vi "SequenceEditor.vi"() -> ()   [LabVIEW 2017]
panel:
  in  "Properties Table":refnum<k24>(container)
  out "IsBusy":bool=TRUE
  out "ExpID":string="Exp967f258c607eed45caf40f4c3101458dC" caption="Exp. ID (Debug)"
  out "Reduced Sequence":dbl[](graph)
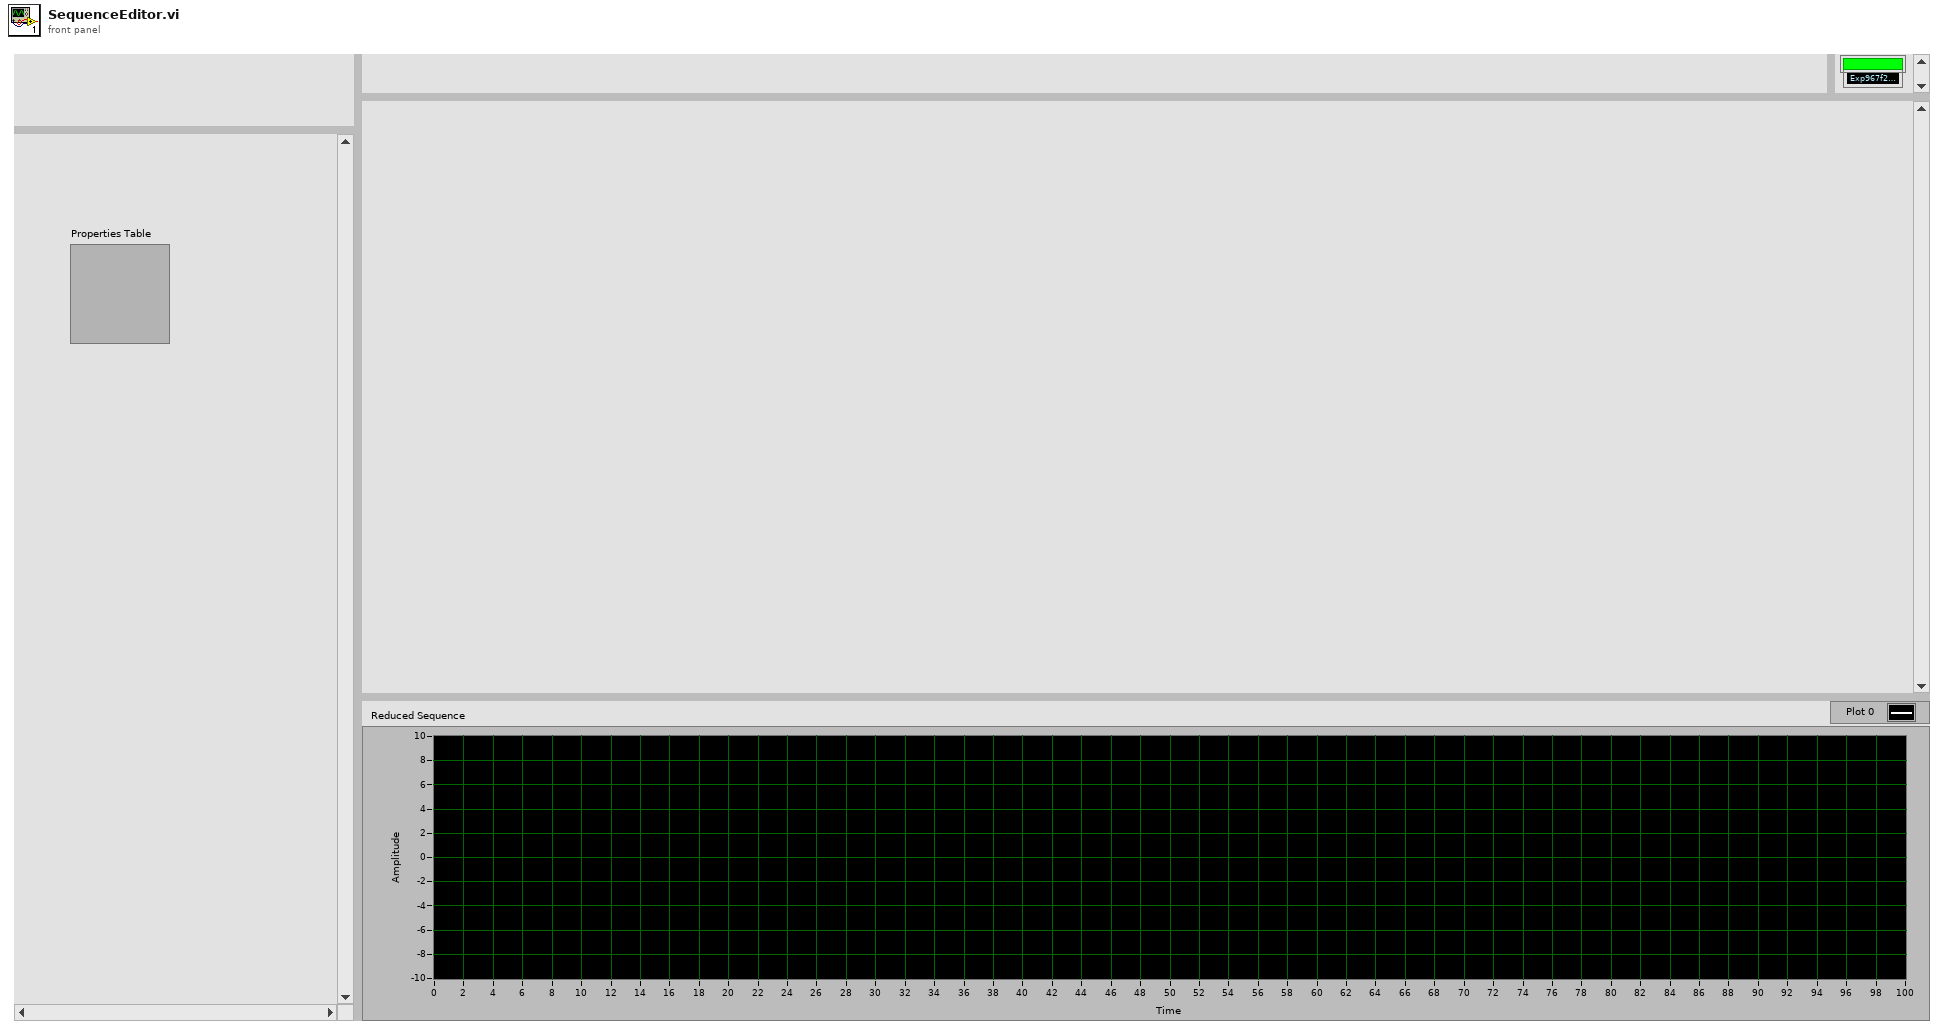
[diagram p1: front panel]
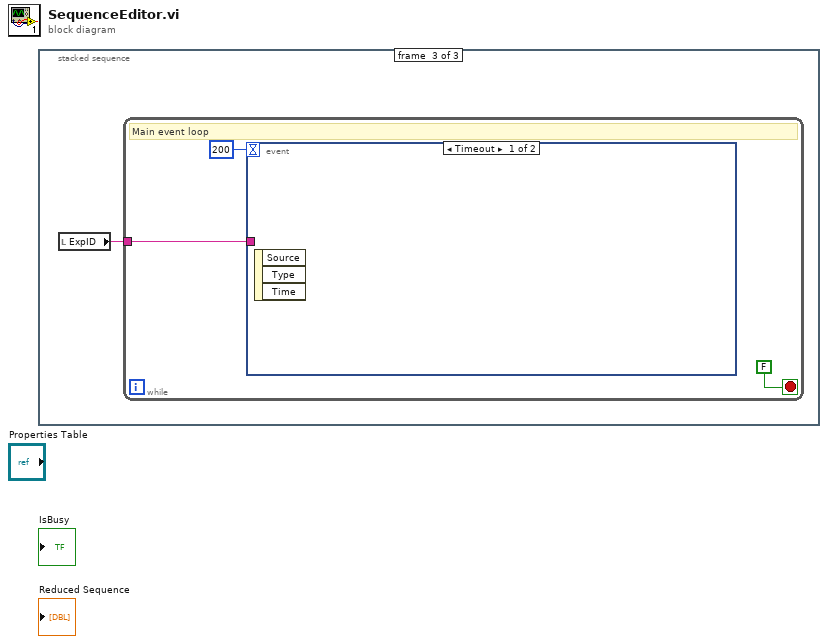
[diagram p0: block diagram]
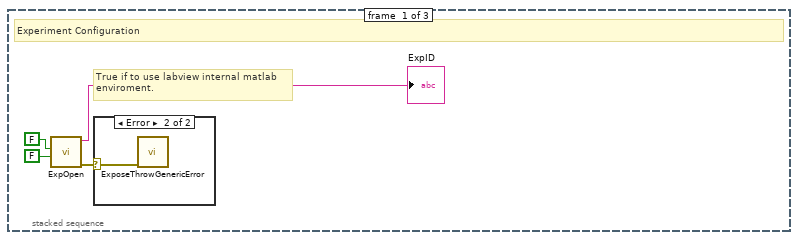
[diagram p2: hidden frame]
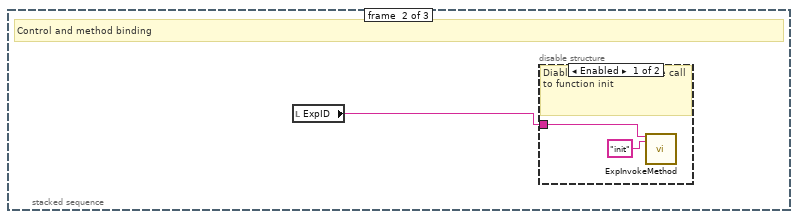
[diagram p4: hidden frame]
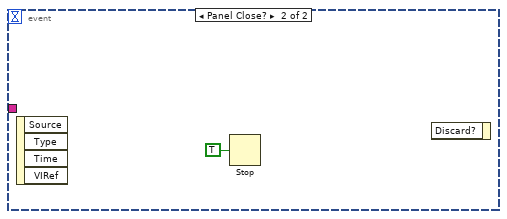
[diagram p6: hidden frame]
diagram:
  n1 = stacked-sequence {
    frame #0 {
      # "True if to use labview internal matlab\nenviroment."
      # "Experiment Configuration"
      n2 = call "ExpOpen.vi"("Do Expose Logging"=FALSE, "Requires Matlab Enviroment"=FALSE) -> ("error out"=w2:errorcluster, "ExpID"=→"ExpID":string)  [unwired: 7 in, 1 out]
      n3 = case shown="Error" w2 {
        selector: w2 -> [_ w5]
        frame No Error {
        }
        frame Error {
          n4 = call "ExposeThrowGenericError.vi"("error in (no error)"=w5) -> ()  [unwired: 10 in, 1 out]
        }
      }
    }
    frame #1 {
      # "Control and method binding"
      n5 = local read "ExpID"() -> (w6:string)
      n6 = disable-structure shown="Enabled" {
        disable-tunnel: w6 -> [w7 _]
        frame Enabled {
          # "Diable this to remove the call to function init"
          n7 = call "ExpInvokeMethod.vi"("ExpID"=w7, "Method Name"="init") -> ()  [unwired: 15 in, 3 out]
        }
        frame Disabled {
        }
      }
    }
    frame #2 {
      n8 = local read "ExpID"() -> (w9:string)
      n9 = while {
        tunnel: w9 -> [w10]
        stop <- FALSE stop-if-true
        # "Main event loop"
        n10 = event shown="[0] Timeout" {
          selector: _ -> [_ _]
          dyn-events: _ -> [_ _]
          timeout: 200 -> [_ _]
          tunnel: w10 -> [_ _]
          event Timeout {
            n11 = event-data() -> ()  [unwired: 1 in, 3 out]
          }
          event Panel Close? {
            n12 = event-data() -> ()  [unwired: 1 in, 4 out]
            n13 = Stop(stop? (T)=TRUE) -> ()
            n14 = event-data() -> ()  [unwired: 2 in, 1 out]
          }
        }
      }
    }
  }
